vi "Set Read Timeout.vi"(8 "error in (no error)":errorcluster, 10 "read operation timeout":i32=5000, 11 "ELAN Master in":refnum<class "ELAN Master.lvclass">) -> (0 "error out":errorcluster, 3 "ELAN Master out":refnum<class "ELAN Master.lvclass">)   [LabVIEW 2021, in "ELAN Master.lvclass"]
doc: "<B>Read Timeout</B> specifies the read operation timeout. You can use a Modbus master instance to perform read operations on a Modbus slave with the specified timeout."
uses:
  ELAN Master.lvclass
  ELAN Master.lvclass/ELAN Master.ctl
  Transmission Data Unit/ELAN/ELAN Data Unit.lvclass/ELAN Data Unit.ctl
  Transmission Data Unit/ELAN/ELAN Data Unit.lvclass
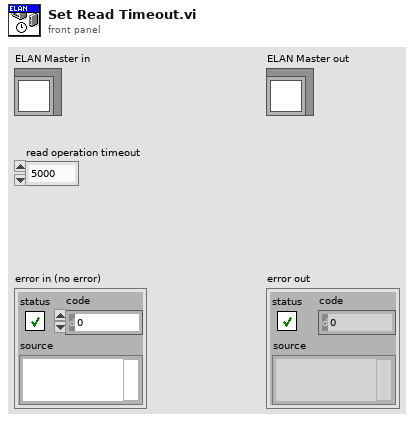
[diagram p1: front panel]
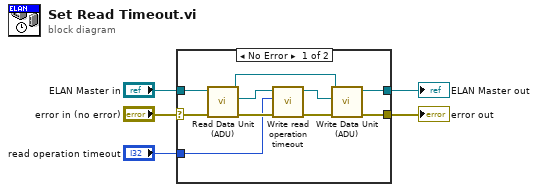
[diagram p0: block diagram]
diagram:
  n1 = case shown="No Error" "error in (no error)" {
    selector: "error in (no error)" -> [w6 w16]
    tunnel: "read operation timeout" -> [w10 _]
    tunnel: [w9 w17] -> w4
    tunnel: "ELAN Master in" -> [w8 w17]
    tunnel: [w7 w16] -> w2
    frame No Error {
      n2 = call "Read Data Unit (ADU).vi"("error in (no error)"=w6, "ELAN Master in"=w8) -> ("error out"=w11:errorcluster, "ASCII Data Unit"=w14:refnum<class "ELAN Data Unit.lvclass">, "ELAN Master out"=w15:refnum<class "ELAN Master.lvclass">)  [unwired: 7 in]
      n3 = call "Write read operation timeout.vi"("error in (no error)"=w11, "read operation timeout"=w10, "ELAN Data Unit in"=w14) -> ("error out"=w12:errorcluster, "ELAN Data Unit out"=w13:refnum<class "ELAN Data Unit.lvclass">)  [unwired: 7 in]
      n4 = call "Write Data Unit (ADU).vi"("error in (no error)"=w12, "ASCII Data Unit"=w13, "ELAN Master in"=w15) -> ("error out"=w7:errorcluster, "ELAN Master out"=w9:refnum<class "ELAN Master.lvclass">)  [unwired: 7 in]
    }
    frame Error {
    }
  }
  "error out" <- w2
  "ELAN Master out" <- w4
